vi "CPP-6068Special.vi"() -> (5 "Plug in titles":string[](array[string]), 7 "Plug in values":string[](array[string]))   [LabVIEW 2014]
uses:
  Globals/Meas_global.vi
  CPP/ProjectSpecific/6068-VeerTowers/MesowestParse/MetDataGlobal.vi
  Globals/Constants_global.vi
panel:
  in  "Include Anemometer Data?":bool=TRUE
  in  "Frequency Band Analysis?":bool=TRUE
  in  "Include Met Data?":bool=TRUE
  out "Results":string[][](table)
  in  "OutputFile":path=path "/TCL-HD/Users/tlawton/Desktop/6068Dump.xls"
  out "BlockStartTime":dbl format="%#_12f"
  in  "SearchBands":cluster{"Min":dbl, "Max":dbl, "Name":string}[](array[cluster])=[{"Min"=40.0, "Max"=70.0, "Name"="60Hz:Band"}, {"Min"=100.0, "Max"=140.0, "Name"="120Hz:Band"}, {"Min"=450.0, "Max"=510.0, "Name"="480Hz:Band"}, {"Min"=600.0, "Max"=680.0, "Name"="640Hz:Band"}, {"Min"=520.0, "Max"=590.0, "Name"="550Hz:Band"}]
  out "TimeRunStarted":dbl format="%^<%H:%M:%S\n%x %Z>T"
  out "Processing last block?":bool
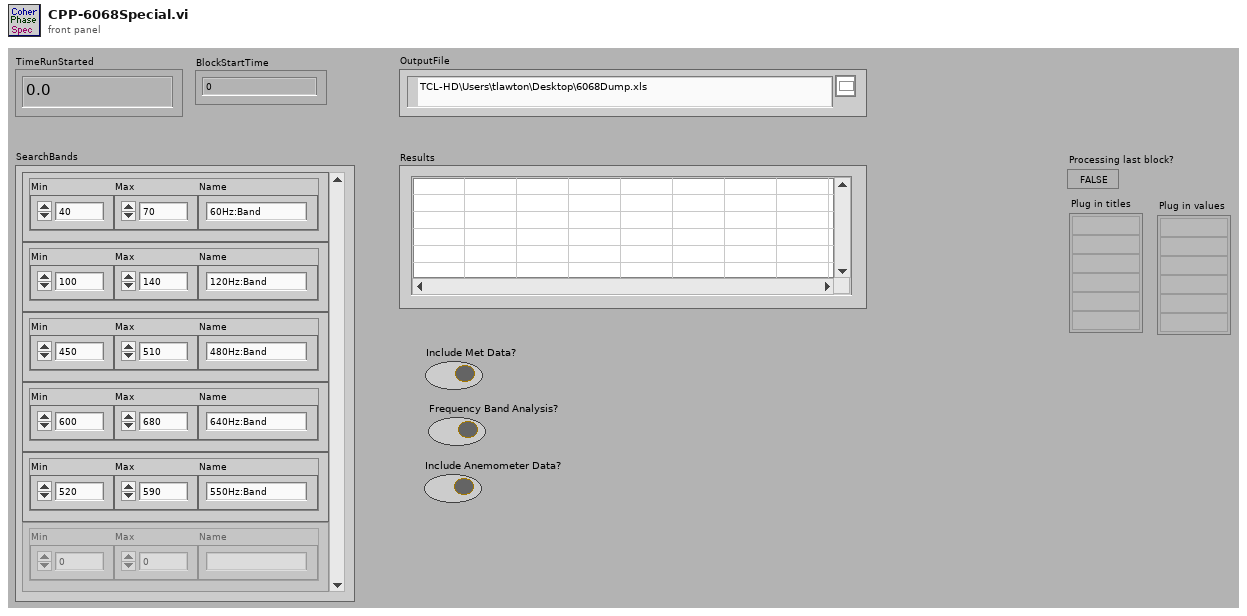
[diagram p1: front panel]
types:
  T1 = enum16{"Overwrite", "Append", "Append and Truncate", "Read", "Lookup"}
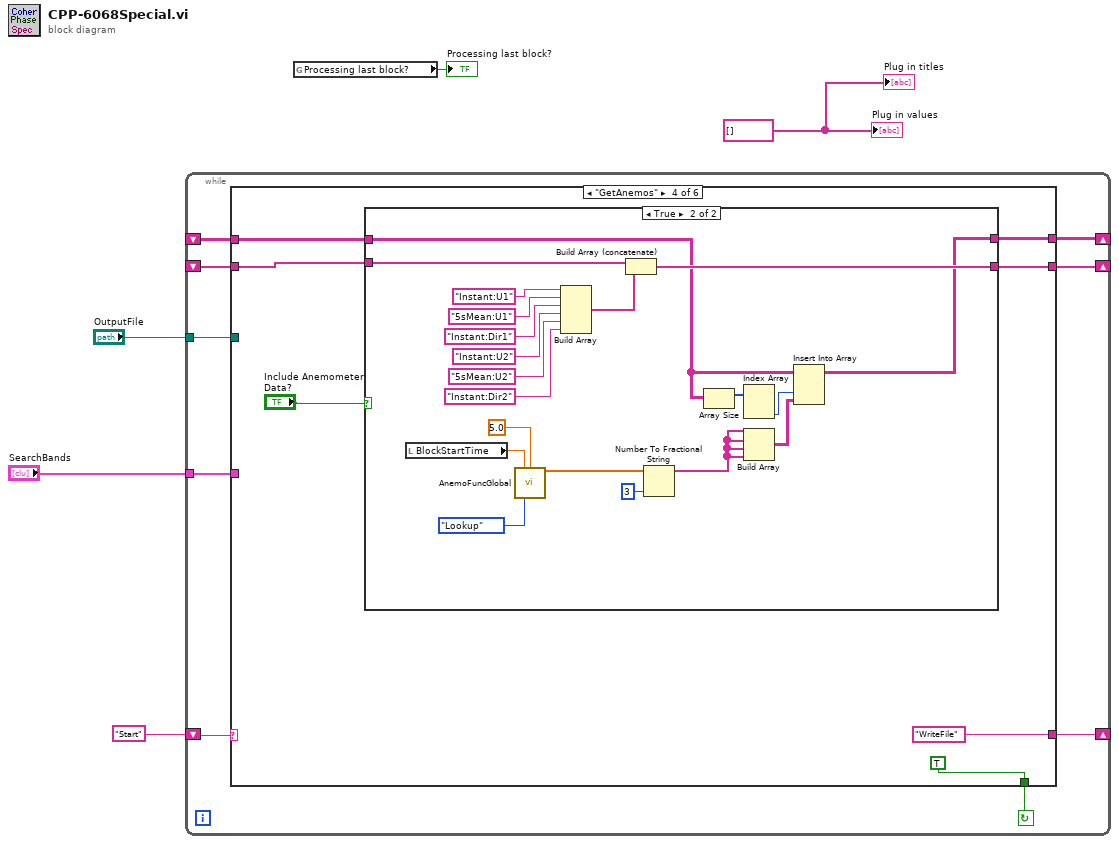
[diagram p0: block diagram]
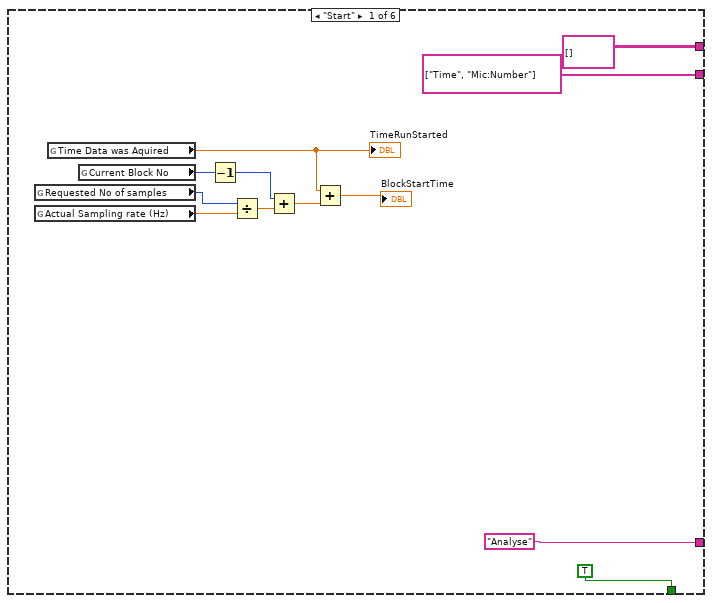
[diagram p2: hidden frame]
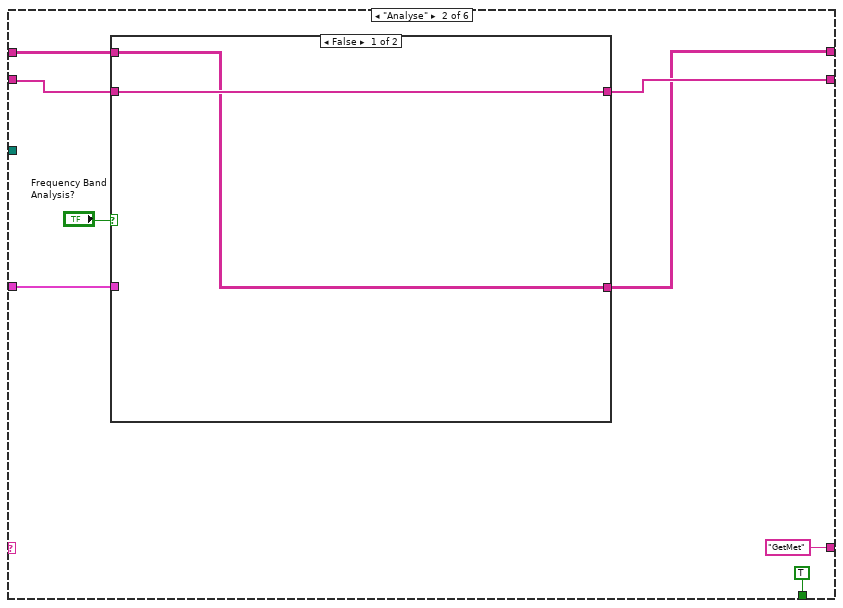
[diagram p3: hidden frame]
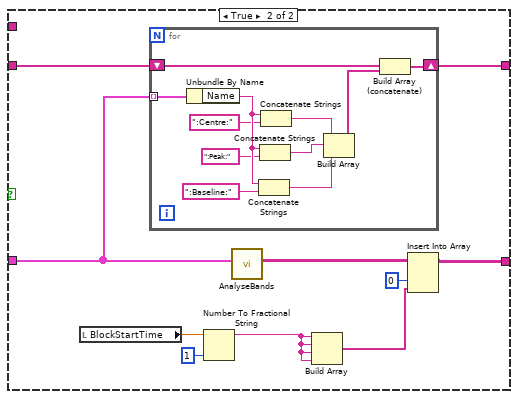
[diagram p4: hidden frame]
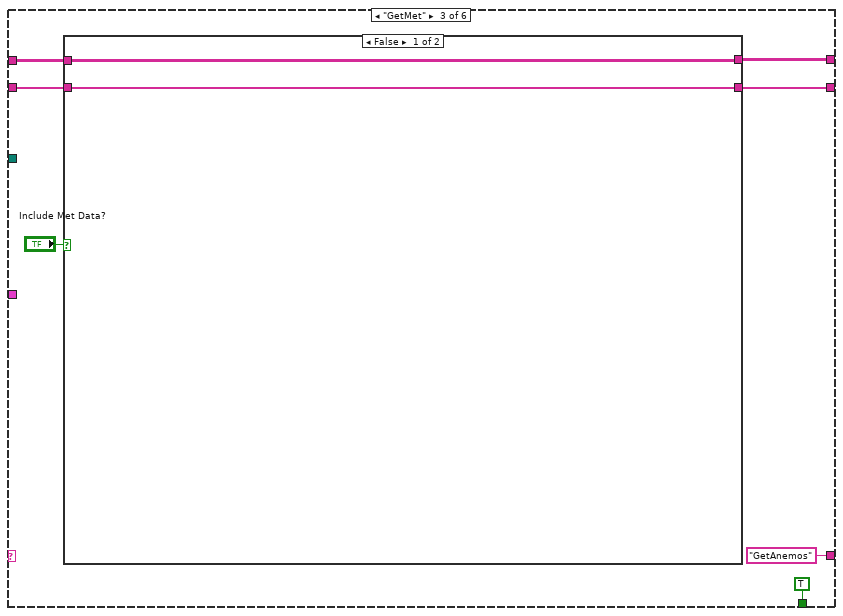
[diagram p5: hidden frame]
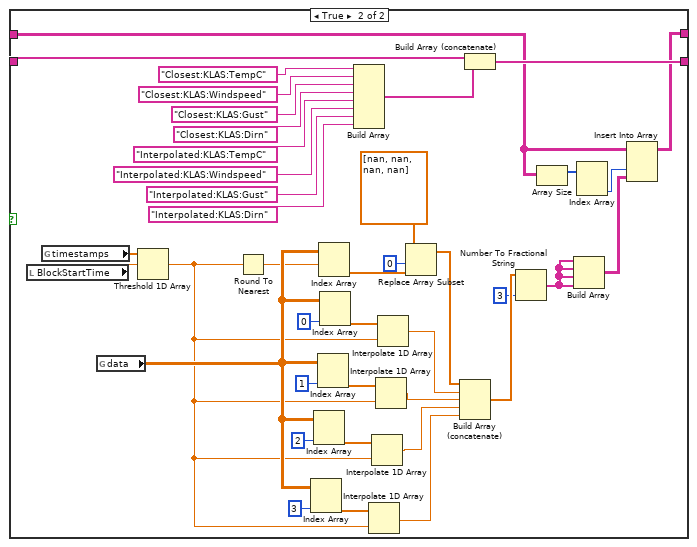
[diagram p6: hidden frame]
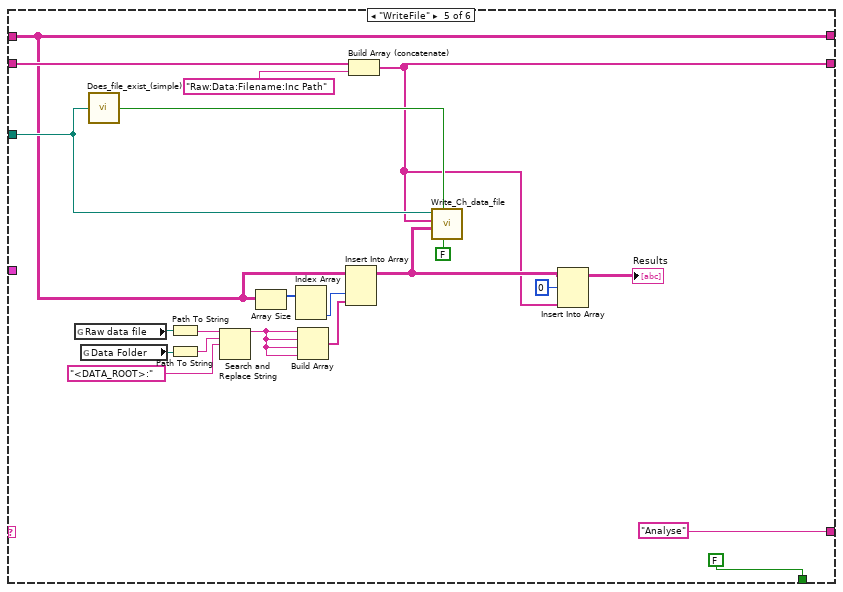
[diagram p8: hidden frame]
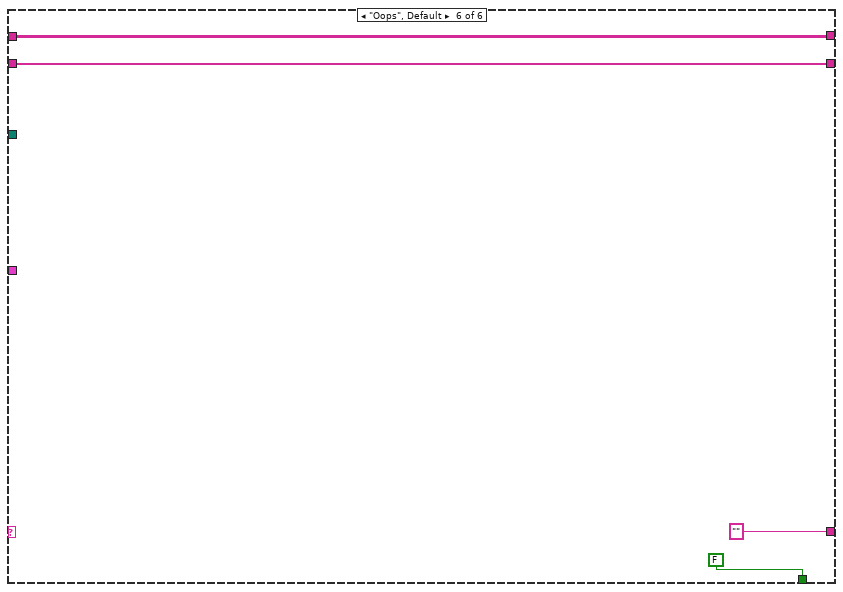
[diagram p9: hidden frame]
diagram:
  w4 = string[] [] ("Add in values")
  n1 = while {
    tunnel: "SearchBands" -> [w14]
    shift-right: [w12] -> _
    shift-left: "Start" -> [w13]
    shift-right: [w9] -> _
    shift-left: _ -> [w10]
    shift-right: [w7] -> _
    shift-left: _ -> [w8]
    tunnel: "OutputFile" -> [w6]
    stop <- w11 continue-if-true
    n2 = case shown="\"GetAnemos\"" w13 {
      tunnel: w14 -> [_ w33 _ _ _ _]
      tunnel: ["Analyse" "GetMet" "GetAnemos" "WriteFile" "Analyse" ""] -> w12
      tunnel: [TRUE TRUE TRUE TRUE FALSE FALSE] -> w11
      tunnel: w10 -> [_ w32 w62 w111 w141 w158]
      tunnel: [string[] ["Time", "Mic:Number"] w31 w61 w110 w139 w158] -> w9
      tunnel: [string[][] [] ("Results") w30 w59 w109 w136 w157] -> w7
      tunnel: w8 -> [_ w28 w60 w108 w136 w157]
      tunnel: w6 -> [_ _ _ _ w143 _]
      frame "Start" {
        n3 = global read "Meas_global.vi" "Requested No of samples"() -> (w24:i32)
        n4 = global read "Meas_global.vi" "Actual Sampling rate (Hz)"() -> (w23:dbl)
        n5 = global read "Meas_global.vi" "Time Data was Aquired"() -> (w19:dbl)
        "TimeRunStarted" <- w19
        n6 = global read "Meas_global.vi" "Current Block No"() -> (w25:i32)
        n7 = Decrement(x=w25) -> (x-1=w21:i32)
        n8 = Divide(x=w24, y=w23) -> (x/y=w22:dbl)
        n9 = Add(x=w21, y=w22) -> (x+y=w20:dbl)
        n10 = Add(x=w19, y=w20) -> (x+y=→"BlockStartTime":dbl)
      }
      frame "Analyse" {
        n11 = case shown="False" "Frequency Band Analysis?" {
          tunnel: w33 -> [_ w42]
          tunnel: w32 -> [w36 w41]
          tunnel: [w36 w40] -> w31
          tunnel: [w35 w39] -> w30
          tunnel: w28 -> [w35 _]
          frame False {
          }
          frame True {
            n12 = local read "BlockStartTime"() -> (w43:dbl)
            n13 = for {
              shift-right: [w49] -> w40
              shift-left: w41 -> [w47]
              tunnel: w42 -> [w57] mode=indexing
              n14 = Unbundle By Name(w57) -> ("Name"=w56:string)
              n15 = Concatenate Strings(w56, ":Baseline:" ("string")) -> (w50:string)
              n16 = Concatenate Strings(w56, ":Peak:" ("string")) -> (w51:string)
              n17 = Concatenate Strings(w56, ":Centre:" ("string")) -> (w52:string)
              n18 = Build Array(w52, w51, w50) -> (w48:string[])
              n19 = Build Array (concatenate)(w47, w48) -> (w49:string[])
            }
            n20 = Number To Fractional String(number=w43, precision (6)=i16 1) -> (F-format string=w38:string)  [unwired: 2 in]
            n21 = call "AnalyseBands.vi"("SearchBands"=w42) -> ("Results"=w46:string[][])  [unwired: 10 in]
            n22 = Build Array(w38, w38, w38, w38) -> (w45:string[])
            n23 = Insert Into Array(array=w46, index (col)=0 ("disabled index (col)"), new element=w45) -> (w39:string[][])  [unwired: 1 in]
          }
        }
      }
      frame "GetMet" {
        n24 = case shown="False" "Include Met Data?" {
          tunnel: w62 -> [w65 w80]
          tunnel: [w65 w79] -> w61
          tunnel: w60 -> [w66 w76]
          tunnel: [w66 w74] -> w59
          frame False {
          }
          frame True {
            n25 = local read "BlockStartTime"() -> (w105:dbl)
            n26 = global read "MetDataGlobal.vi" "timestamps"() -> (w106:dbl[])
            n27 = global read "MetDataGlobal.vi" "data"() -> (w92:dbl[][])
            n28 = Threshold 1D Array(2:w105, 3:w106) -> (0:w91:dbl)  [unwired: 1 in]
            n29 = Round To Nearest(number=w91) -> (nearest integer value=w90:dbl)
            n30 = Index Array(array=w92, index (col)=3 ("disabled index (col)")) -> (element=w98:dbl[])  [unwired: 1 in]
            n31 = Index Array(array=w92, index (col)=2 ("disabled index (col)")) -> (element=w99:dbl[])  [unwired: 1 in]
            n32 = Index Array(array=w92, index (col)=1 ("disabled index (col)")) -> (element=w102:dbl[])  [unwired: 1 in]
            n33 = Index Array(array=w92, index (row)=w90) -> (element=w71:dbl[])  [unwired: 1 in]
            n34 = Index Array(array=w92, index (col)=0 ("disabled index (col)")) -> (element=w103:dbl[])  [unwired: 1 in]
            n35 = Build Array("Closest:KLAS:TempC", "Closest:KLAS:Windspeed", "Closest:KLAS:Gust", "Closest:KLAS:Dirn", "Interpolated:KLAS:TempC", "Interpolated:KLAS:Windspeed", "Interpolated:KLAS:Gust", "Interpolated:KLAS:Dirn") -> (w81:string[])
            n36 = Interpolate 1D Array(1:w91, 2:w98) -> (0:w93:dbl)
            n37 = Interpolate 1D Array(1:w91, 2:w99) -> (0:w94:dbl)
            n38 = Interpolate 1D Array(1:w91, 2:w102) -> (0:w95:dbl)
            n39 = Interpolate 1D Array(1:w91, 2:w103) -> (0:w96:dbl)
            n40 = Replace Array Subset(array=dbl[] [nan, nan, nan, nan], new element=w71, index=0) -> (w72:dbl[])
            n41 = Build Array (concatenate)(w72, w96, w95, w94, w93) -> (w78:dbl[])
            n42 = Build Array (concatenate)(w80, w81) -> (w79:string[])
            n43 = Number To Fractional String(number=w78, precision (6)=i16 3) -> (F-format string=w67:string[])  [unwired: 2 in]
            n44 = Array Size(array=w76) -> (size(s)=w75:i32[])
            n45 = Build Array(w67, w67, w67, w67) -> (w77:string[][])
            n46 = Index Array(array=w75) -> (element #2=w73:i32)  [unwired: 2 in, 1 out]
            n47 = Insert Into Array(array=w76, index (col)=w73, new element=w77) -> (w74:string[][])  [unwired: 1 in]
          }
        }
      }
      frame "GetAnemos" {
        n48 = case shown="True" "Include Anemometer Data?" {
          tunnel: w111 -> [w114 w128]
          tunnel: [w114 w127] -> w110
          tunnel: [w115 w124] -> w109
          tunnel: w108 -> [w115 w123]
          frame False {
          }
          frame True {
            n49 = local read "BlockStartTime"() -> (w122:dbl)
            n50 = call "AnemoFuncGlobal.vi"("searchValue"=w122, "history(samples)"=5.0 ("fractional index or x"), "Mode"=T1."Lookup") -> ("results"=w120:dbl[])  [unwired: 11 in, 1 out]
            n51 = Build Array("Instant:U1", "5sMean:U1", "Instant:Dir1", "Instant:U2", "5sMean:U2", "Instant:Dir2") -> (w129:string[])
            n52 = Build Array (concatenate)(w128, w129) -> (w127:string[])
            n53 = Number To Fractional String(number=w120, precision (6)=i16 3) -> (F-format string=w118:string[])  [unwired: 2 in]
            n54 = Array Size(array=w123) -> (size(s)=w126:i32[])
            n55 = Index Array(array=w126) -> (element #2=w125:i32)  [unwired: 2 in, 1 out]
            n56 = Build Array(w118, w118, w118, w118) -> (w119:string[][])
            n57 = Insert Into Array(array=w123, index (col)=w125, new element=w119) -> (w124:string[][])  [unwired: 1 in]
          }
        }
      }
      frame "WriteFile" {
        n58 = global read "Meas_global.vi" "Raw data file"() -> (w149:path)
        n59 = global read "Constants_global.vi" "Data Folder"() -> (w148:path)
        n60 = call "Does_file_exist_(simple).vi"("Pathname"=w143) -> ("exists?"=w154:bool)
        n61 = Path To String(path=w149) -> (string=w147:string)
        n62 = Path To String(path=w148) -> (string=w146:string)
        n63 = Search and Replace String(input string=w147, search string=w146, replace string="<DATA_ROOT>:" ("replace string (\"\")")) -> (result string=w145:string)  [unwired: 5 in, 3 out]
        n64 = Array Size(array=w136) -> (size(s)=w151:i32[])
        n65 = Index Array(array=w151) -> (element #2=w150:i32)  [unwired: 2 in, 1 out]
        n66 = Build Array(w145, w145, w145, w145) -> (w152:string[])
        n67 = Insert Into Array(array=w136, index (col)=w150, new element=w152) -> (w140:string[][])  [unwired: 1 in]
        n68 = Build Array (concatenate)(w141, "Raw:Data:Filename:Inc Path") -> (w139:string[])
        n69 = call "Write_Ch_data_file.vi"("Lock File"=FALSE, "exists?"=w154, "Channel Values"=w140, "Channel names"=w139, "Filename"=w143) -> ()  [unwired: 7 in]
        n70 = Insert Into Array(array=w140, index (row)=0, new element=w139) -> (→"Results":string[][])  [unwired: 1 in]
      }
      frame "Oops", Default {
      }
    }
  }
  n71 = global read "Meas_global.vi" "Processing last block?"() -> (→"Processing last block?":bool)
  "Plug in titles" <- w4
  "Plug in values" <- w4
